vi "xijk_norm.vi"(10 "y":sgl[](array[numeric]), 11 "x":i16[](array[numeric])) -> (2 "y_out":sgl[](array[numeric]), 3 "x_out":i16[](array[numeric]))   [LabVIEW 2009]
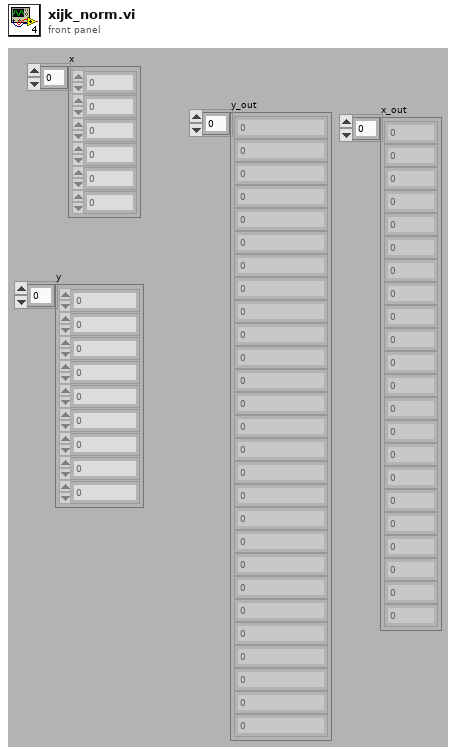
[diagram p1: front panel]
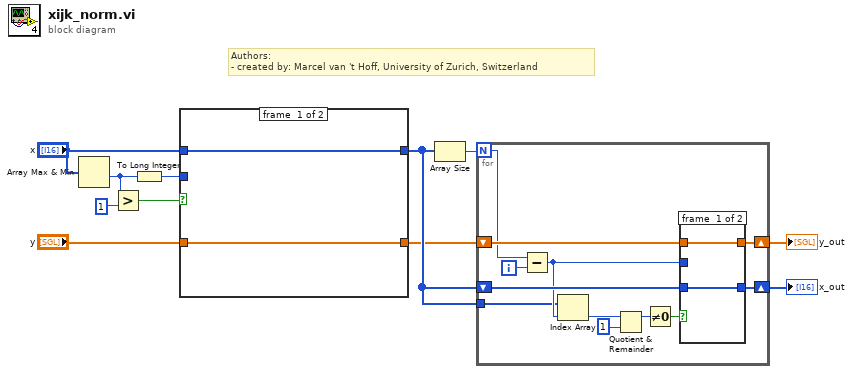
[diagram p0: block diagram]
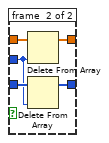
[diagram p2: hidden frame]
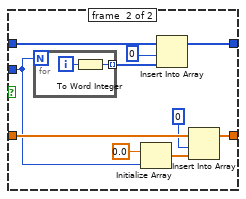
[diagram p3: hidden frame]
diagram:
  # "Authors: \n- created by: Marcel van 't Hoff, University of Zurich, Switzerland"
  n1 = Array Max & Min(array="x") -> (min value=w7:i16)  [unwired: 3 out]
  n2 = Greater?(x=w7, y=i16 1) -> (0:w11:bool)
  n3 = To Long Integer(number=w7) -> (32bit integer=w1:i32)
  n4 = case shown="True" w11 {
    tunnel: "y" -> [w13 w20]
    tunnel: "x" -> [w12 w22]
    tunnel: w1 -> [_ w16]
    tunnel: [w12 w14] -> w3
    tunnel: [w13 w17] -> w2
    frame #0 {
    }
    frame #1 {
      n5 = for {
        N: w16 -> [_]
        tunnel: [w24] -> w15 mode=indexing
        i -> [w25]
        n6 = To Word Integer(number=w25) -> (16bit integer=w24:i16)
      }
      n7 = Initialize Array(sgl 0.0 ("élément"), w16) -> (w19:sgl[])
      n8 = Insert Into Array(array=w22, index=0 ("indice"), new element=w15) -> (w14:i16[])
      n9 = Insert Into Array(array=w20, index=0 ("indice"), new element=w19) -> (w17:sgl[])
    }
  }
  n10 = Array Size(array=w3) -> (size(s)=w4:i32)
  n11 = for {
    N: w4 -> [w30]
    tunnel: w3 -> [w27]
    shift-right: [w36] -> w6
    shift-left: w2 -> [w34]
    shift-right: [w37] -> w5
    shift-left: w3 -> [w35]
    i -> [w29]
    n12 = Subtract(x=w30, y=w29) -> (x-y=w28:i32)
    n13 = Index Array(array=w27, index=w28) -> (element=w26:i16)
    n14 = Quotient & Remainder(x=w26, y=i16 1) -> (x-y*floor(x/y)=w32:i16)  [unwired: 1 out]
    n15 = Not Equal To 0?(x=w32) -> (x != 0?=w31:bool)
    n16 = case shown="True" w31 {
      tunnel: w35 -> [w39 w44]
      tunnel: w28 -> [_ w43]
      tunnel: [w38 w42] -> w36
      tunnel: [w39 w41] -> w37
      tunnel: w34 -> [w38 w40]
      frame #0 {
      }
      frame #1 {
        n17 = Delete From Array(array=w40, index=w43) -> (array with subset deleted=w42:sgl[])  [unwired: 1 in, 1 out]
        n18 = Delete From Array(array=w44, index=w43) -> (array with subset deleted=w41:i16[])  [unwired: 1 in, 1 out]
      }
    }
  }
  "x_out" <- w5
  "y_out" <- w6
